vi "EQE_DataConvert.vi"(9 "Input":cluster{"Wavelength":dbl, "Lock-in R":dbl}, 10 "Calibration":bool=TRUE, 11 "Detector":enum16{"Silicon", "Germanium", "InGaAs"}(ring)) -> (1 "Output":cluster{"Wavelength":dbl, "EQE":dbl})   [LabVIEW 2017]
uses:
  <vilib>/Utility/file.llb/Read Delimited Spreadsheet (DBL).vi
  <vilib>/Utility/file.llb/Write Delimited Spreadsheet (DBL).vi
panel:
  out "Intensity (New cal factor)":dbl
  out "Output array":dbl[][](array[numeric])
  out "Detector EQE":dbl[][](array[numeric])
  out "Input array":dbl[][](array[numeric])
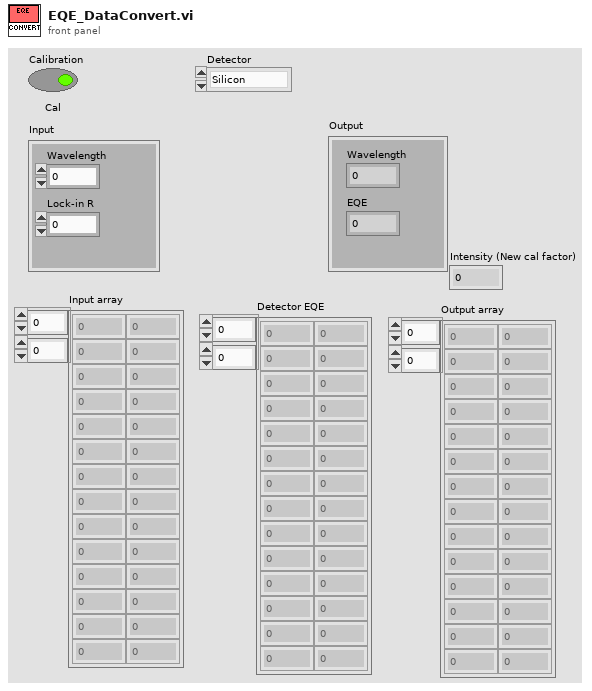
[diagram p1: front panel]
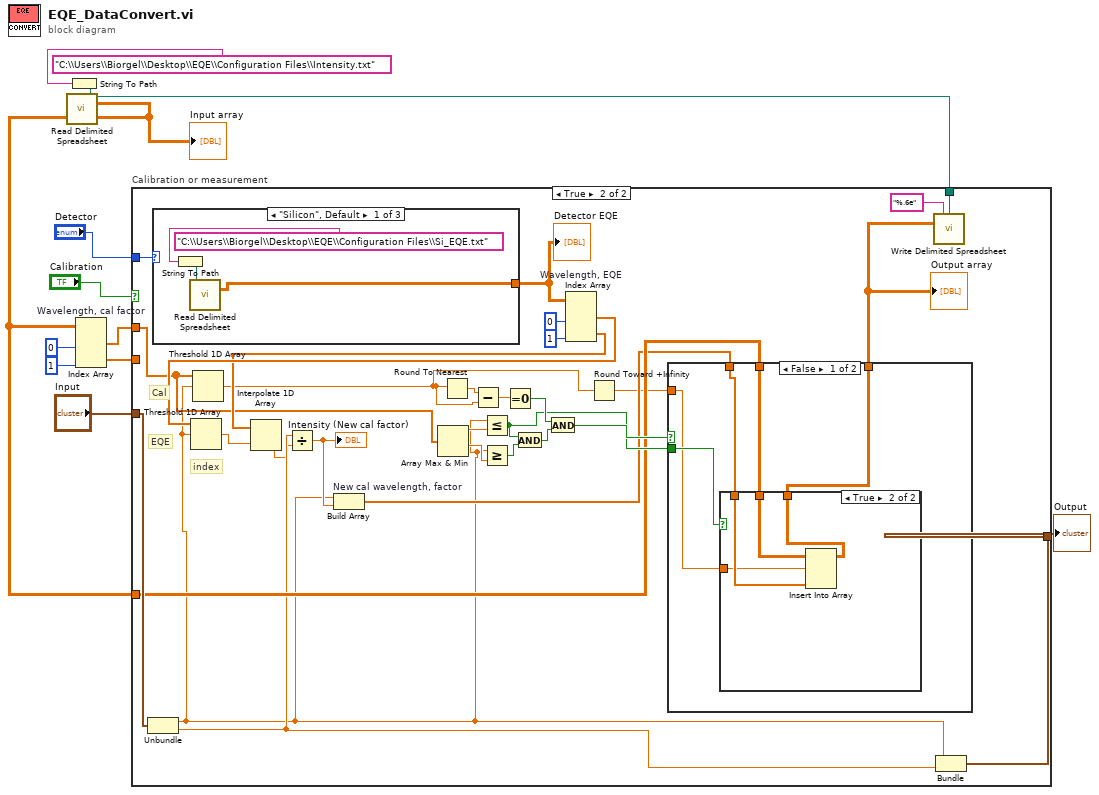
[diagram p0: block diagram]
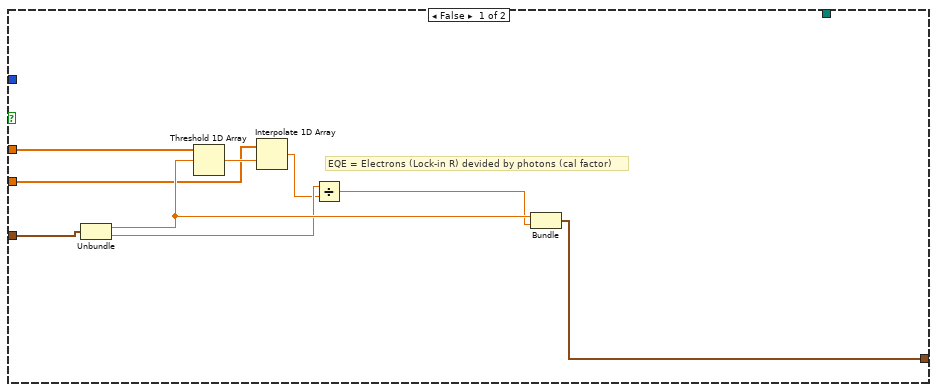
[diagram p2: hidden frame]
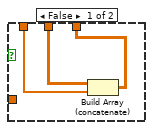
[diagram p3: hidden frame]
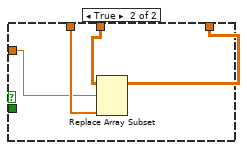
[diagram p4: hidden frame]
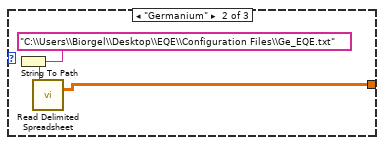
[diagram p5: hidden frame]
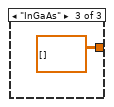
[diagram p6: hidden frame]
diagram:
  n1 = String To Path(string="C:\\Users\\Biorgel\\Desktop\\EQE\\Configuration Files\\Intensity.txt") -> (path=w7:path)
  n2 = call-poly <vilib>:"Read Delimited Spreadsheet.vi"("file path (dialog if empty)"=w7) -> ("new file path (Not A Path if cancelled)"=w6:path, "all rows"=w1:dbl[][])  [unwired: 9 in, 4 out]
  "Input array" <- w1
  n3 = Index Array "Wavelength, cal factor"(array=w1, index (col) #1=0 ("disabled index (col)"), index (col) #2=1 ("index (col)")) -> (element #1=w3:dbl[], element #2=w2:dbl[])  [unwired: 2 in]
  n4 = case "Calibration or measurement" shown="True" "Calibration" {
    tunnel: "Input" -> [w21 w51]
    tunnel: [w20 w50] -> w11
    tunnel: "Detector" -> [_ w48]
    tunnel: w6 -> [_ w49]
    tunnel: w3 -> [w16 w34]
    tunnel: w2 -> [w15 _]
    tunnel: w1 -> [_ w30]
    frame False {
      # "EQE = Electrons (Lock-in R) devided by photons (cal factor)"
      n5 = Unbundle(w21) -> ("Wavelength"=w18:dbl, "Lock-in R"=w14:dbl)
      n6 = Threshold 1D Array(2:w18, 3:w16) -> (0:w19:dbl)  [unwired: 1 in]
      n7 = Interpolate 1D Array(1:w19, 2:w15) -> (0:w13:dbl)
      n8 = Divide(x=w14, y=w13) -> (x/y=w17:dbl)
      n9 = Bundle("Wavelength"=w18, w17) -> (w20:cluster{"Wavelength":dbl, dbl})  [unwired: 1 in]
    }
    frame True {
      # "index"
      # "EQE"
      # "Cal"
      n10 = Unbundle(w51) -> ("Wavelength"=w23:dbl, "Lock-in R"=w25:dbl)
      n11 = case shown="\"Silicon\", Default" w48 {
        tunnel: [w68 w71 dbl[][] [] ("all rows")] -> w47
        frame "Silicon", Default {
          n12 = String To Path(string="C:\\Users\\Biorgel\\Desktop\\EQE\\Configuration Files\\Si_EQE.txt") -> (path=w70:path)
          n13 = call-poly <vilib>:"Read Delimited Spreadsheet.vi"("file path (dialog if empty)"=w70) -> ("all rows"=w68:dbl[][])  [unwired: 9 in, 5 out]
        }
        frame "Germanium" {
          n14 = String To Path(string="C:\\Users\\Biorgel\\Desktop\\EQE\\Configuration Files\\Ge_EQE.txt") -> (path=w73:path)
          n15 = call-poly <vilib>:"Read Delimited Spreadsheet.vi"("file path (dialog if empty)"=w73) -> ("all rows"=w71:dbl[][])  [unwired: 9 in, 5 out]
        }
        frame "InGaAs" {
        }
      }
      "Detector EQE" <- w47
      n16 = Threshold 1D Array(2:w23, 3:w34) -> (0:w26:dbl)  [unwired: 1 in]
      n17 = Array Max & Min(array=w34) -> (max value=w39:dbl, min value=w38:dbl)  [unwired: 2 out]
      n18 = Round To Nearest(number=w26) -> (nearest integer value=w40:dbl)
      n19 = Subtract(x=w40, y=w26) -> (x-y=w41:dbl)
      n20 = Less Or Equal?(x=w23, y=w39) -> (x <= y?=w32:bool)
      n21 = Greater Or Equal?(x=w23, y=w38) -> (x >= y?=w35:bool)
      n22 = Equal To 0?(x=w41) -> (x = 0?=w37:bool)
      n23 = And(x=w32, y=w35) -> (x .and. y?=w36:bool)
      n24 = And(x=w37, y=w36) -> (x .and. y?=w33:bool)
      n25 = Index Array "Wavelength, EQE"(array=w47, index (col) #1=0 ("disabled index (col)"), index (col) #2=1 ("index (col)")) -> (element #1=w44:dbl[], element #2=w42:dbl[])  [unwired: 2 in]
      n26 = Threshold 1D Array(2:w23, 3:w44) -> (0:w43:dbl)  [unwired: 1 in]
      n27 = Interpolate 1D Array(1:w43, 2:w42) -> (0:w24:dbl)
      n28 = Divide(x=w25, y=w24) -> (x/y=w29:dbl)
      "Intensity (New cal factor)" <- w29
      n29 = Build Array "New cal wavelength, factor"(w23, w29) -> (w28:dbl[])
      n30 = Round Toward +Infinity(x=w26) -> (ceil(x): smallest int >= x=w27:dbl)
      n31 = case shown="False" w33 {
        tunnel: w30 -> [w55 w67]
        tunnel: w28 -> [w54 w66]
        tunnel: [w53 w65] -> w31
        tunnel: w32 -> [w56 _]
        tunnel: w27 -> [w52 w64]
        frame False {
          n32 = case shown="True" w56 {
            tunnel: [w57 w63] -> w53
            tunnel: w55 -> [w59 w62]
            tunnel: w54 -> [w58 w61]
            tunnel: w52 -> [_ w60]
            frame False {
              n33 = Build Array (concatenate)(w59, w58) -> (w57:dbl[][])
            }
            frame True {
              n34 = Insert Into Array(array=w62, index (row)=w60, new element=w61) -> (w63:dbl[][])  [unwired: 1 in]
            }
          }
        }
        frame True {
          n35 = Replace Array Subset(array=w67, new element=w66, index (row)=w64) -> (w65:dbl[][])  [unwired: 1 in]
        }
      }
      "Output array" <- w31
      n36 = call-poly <vilib>:"Write Delimited Spreadsheet.vi"("file path (dialog if empty)"=w49, "format (%.3f)"="%.6e", "2D data"=w31) -> ()  [unwired: 11 in, 2 out]
      n37 = Bundle("Wavelength"=w23, "Lock-in R"=w25) -> (w50:cluster{"Wavelength":dbl, "Lock-in R":dbl})  [unwired: 1 in]
    }
  }
  "Output" <- w11
